vi "CRYGet dBref NewUnit.vi"(8 "New dB ref in":dbl, 10 "Old dB ref in":dbl, 11 "Unit in":string) -> (2 "Out New Unit":string)   [LabVIEW 2013]
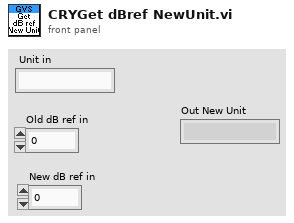
[diagram p1: front panel]
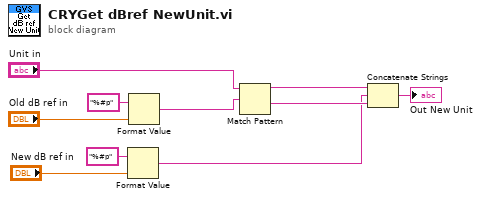
[diagram p0: block diagram]
diagram:
  n1 = Format Value(format string="%#p", value (0)="New dB ref in") -> (output string=w3:string)  [unwired: 1 in]
  n2 = Format Value(format string="%#p", value (0)="Old dB ref in") -> (output string=w7:string)  [unwired: 1 in]
  n3 = Match Pattern(string="Unit in", regular expression=w7) -> (before substring=w5:string, after substring=w4:string)  [unwired: 3 out]
  n4 = Concatenate Strings(w5, w3, w4) -> (→"Out New Unit":string)
